vi "Configure Voltage Sweep.vi"(0 "VISA resource name":refnum<visa-resource-name>, 1 "Voltage Sweep Delay (1s)":dbl=1.0, 2 "Autoconfig Arm (T: Enable)":bool=TRUE, 5 "Voltage Sweep Start (0V)":dbl, 7 "Voltage Sweep Stop (10V)":dbl=10.0, 9 "Voltage Sweep Step Size (1V)":dbl=1.0, 11 "error in (no error)":errorcluster) -> (4 "VISA resource name out":refnum<visa-resource-name>, 15 "error out":errorcluster)   [LabVIEW 2021, in "Keithley 648X Series.lvlib"]
doc: "Configures the voltage sweep function.\n\n<b>Note:</b>\nThis supports Model 6487 only"
uses:
  <instrlib>/Keithley 648X Series/Keithley 648X Series.lvlib
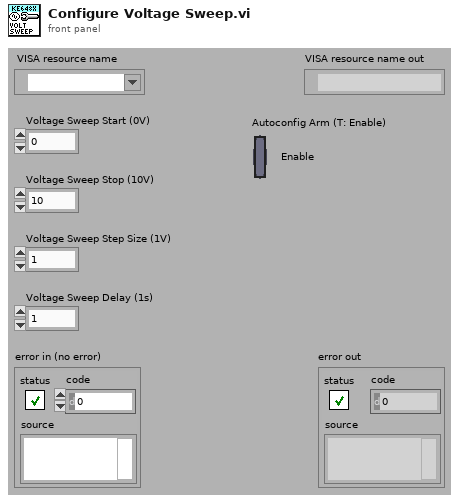
[diagram p1: front panel]
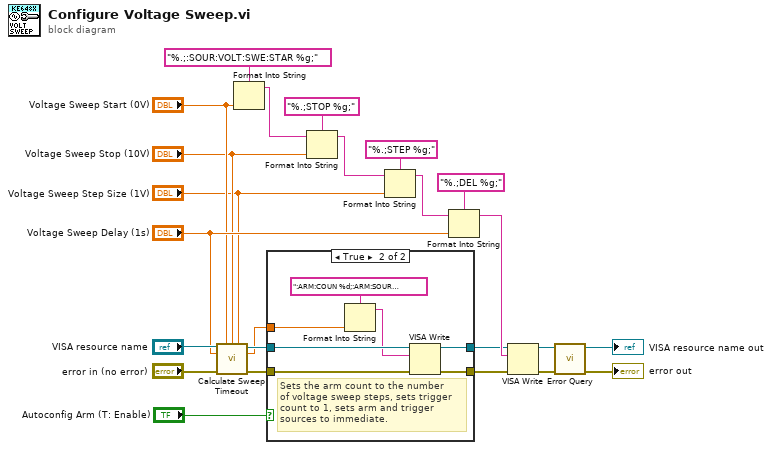
[diagram p0: block diagram]
diagram:
  n1 = call <instrlib>:"Calculate Sweep Timeout.vi"("VISA resource name"="VISA resource name", "Voltage Sweep Start (0V)"="Voltage Sweep Start (0V)", "Voltage Sweep Stop (10V)"="Voltage Sweep Stop (10V)", "Voltage Sweep Step Size (1V)"="Voltage Sweep Step Size (1V)", "Voltage Sweep Delay (1s)"="Voltage Sweep Delay (1s)", "error in (no error)"="error in (no error)") -> ("VISA resource name out"=w3:refnum<visa-resource-name>, "Steps"=w1:dbl, "error out"=w2:errorcluster)  [unwired: 7 in]
  n2 = Format Into String(format string="%.;:SOUR:VOLT:SWE:STAR %g;", "Voltage Sweep Start (0V)") -> (resulting string=w18:string)  [unwired: 2 in, 1 out]
  n3 = case shown="True" "Autoconfig Arm (T: Enable)" {
    tunnel: [w26 w33] -> w5
    tunnel: [w25 w32] -> w4
    tunnel: w3 -> [w26 w31]
    tunnel: w2 -> [w25 w30]
    tunnel: w1 -> [_ w28]
    frame False {
    }
    frame True {
      # "Sets the arm count to the number\nof voltage sweep steps, sets trigger \ncount to 1, sets arm and trigger \nsources to immediate."
      n4 = Format Into String(format string=":ARM:COUN %d;:ARM:SOUR IMM;:TRIG:COUN 1;:TRIG:SOUR IMM;", w28) -> (resulting string=w27:string)  [unwired: 2 in, 1 out]
      n5 = VISA Write(VISA resource name=w31, write buffer=w27, error in (no error)=w30) -> (VISA resource name out=w33:refnum<visa-resource-name>, error out=w32:errorcluster)  [unwired: 1 out]
    }
  }
  n6 = Format Into String(format string="%.;STOP %g;", initial string=w18, "Voltage Sweep Stop (10V)") -> (resulting string=w16:string)  [unwired: 1 in, 1 out]
  n7 = Format Into String(format string="%.;STEP %g;", initial string=w16, "Voltage Sweep Step Size (1V)") -> (resulting string=w15:string)  [unwired: 1 in, 1 out]
  n8 = Format Into String(format string="%.;DEL %g;", initial string=w15, "Voltage Sweep Delay (1s)") -> (resulting string=w13:string)  [unwired: 1 in, 1 out]
  n9 = VISA Write(VISA resource name=w5, write buffer=w13, error in (no error)=w4) -> (VISA resource name out=w22:refnum<visa-resource-name>, error out=w21:errorcluster)  [unwired: 1 out]
  n10 = call <instrlib>:"Error Query.vi"("error in (no error)"=w21, "VISA resource name"=w22) -> ("error out"=→"error out":errorcluster, "VISA resource name out"=→"VISA resource name out":refnum<visa-resource-name>)  [unwired: 6 in, 2 out]
